vi "Get Hardware Channel Data (Rx or Tx).vi"(7 "direction":T11, 8 "error in":errorcluster, 11 "custom device ref in":T9 format="%.0x") -> (0 "error out":errorcluster, 2 "hardware channel data":T1[](array[typedef]) {"labels settings for RT"."Label Timestamp Channel Data Reference" format="%.0x"; "labels settings for RT"."Word Initial Raw Value" format="%032.0f"; "labels settings for RT"."Label Disable/Trigger Channel Reference" format="%.0x"; "labels settings for RT"."parameter driver data"."Tx parameter refs" format="%.0x"; "labels settings for RT"."parameter driver data"."Rx block data refs"."Data Reference" format="%.0x"; "labels settings for RT"."SDI" format="%02b"; "labels settings for RT"."label" format="%.0o"}, 3 "custom device ref out":T9 format="%.0x")   [LabVIEW 2020, in "Ballard ARINC 429 Shared.lvlib"]
uses:
  Ballard ARINC 429 Shared.lvlib
  <vilib>/NI VeriStand/Custom Device API/Custom Device API.lvlib
  Custom Device Support/Scripting/Communication Bus Template Scripting.lvlib
  <vilib>/NI VeriStand/Custom Device Tools/Custom Device Utility Library/Custom Device Utility Library.lvlib
  Custom Device Support/Scripting/Constants.vi
  <vilib>/NI VeriStand/Custom Device Tools/Custom Device Utility Library/NI VeriStand - Search for Item by GUID.vi
  <vilib>/NI VeriStand/Custom Device API/Data Access Type.ctl
  <vilib>/NI VeriStand/Custom Device API/Custom Device Item Ref.ctl
  <vilib>/NI VeriStand/Custom Device Tools/Custom Device Utility Library/NI VeriStand - Search for All Items by GUID.vi
  Label.ctl
  Encoding and Decoding/Encoding.ctl
  Encoding and Decoding/Encoding and Decoding.lvlib
  Protocol/Implementations/ARINC429/Parameter Definition.ctl
  Protocol/Implementations/ARINC429/ARINC 429.lvclass
  <vilib>/NI VeriStand/Custom Device API/Data Reference.ctl
  <vilib>/NI VeriStand/Custom Device API/Block Data Reference.ctl
  RT Parameters.ctl
  Transfer Type.ctl
  RT Label Settings.ctl
  RT Hardware Channel Settings.ctl
  <vilib>/NI VeriStand/Custom Device API/Get Item Property (U16).vi
  Direction.ctl
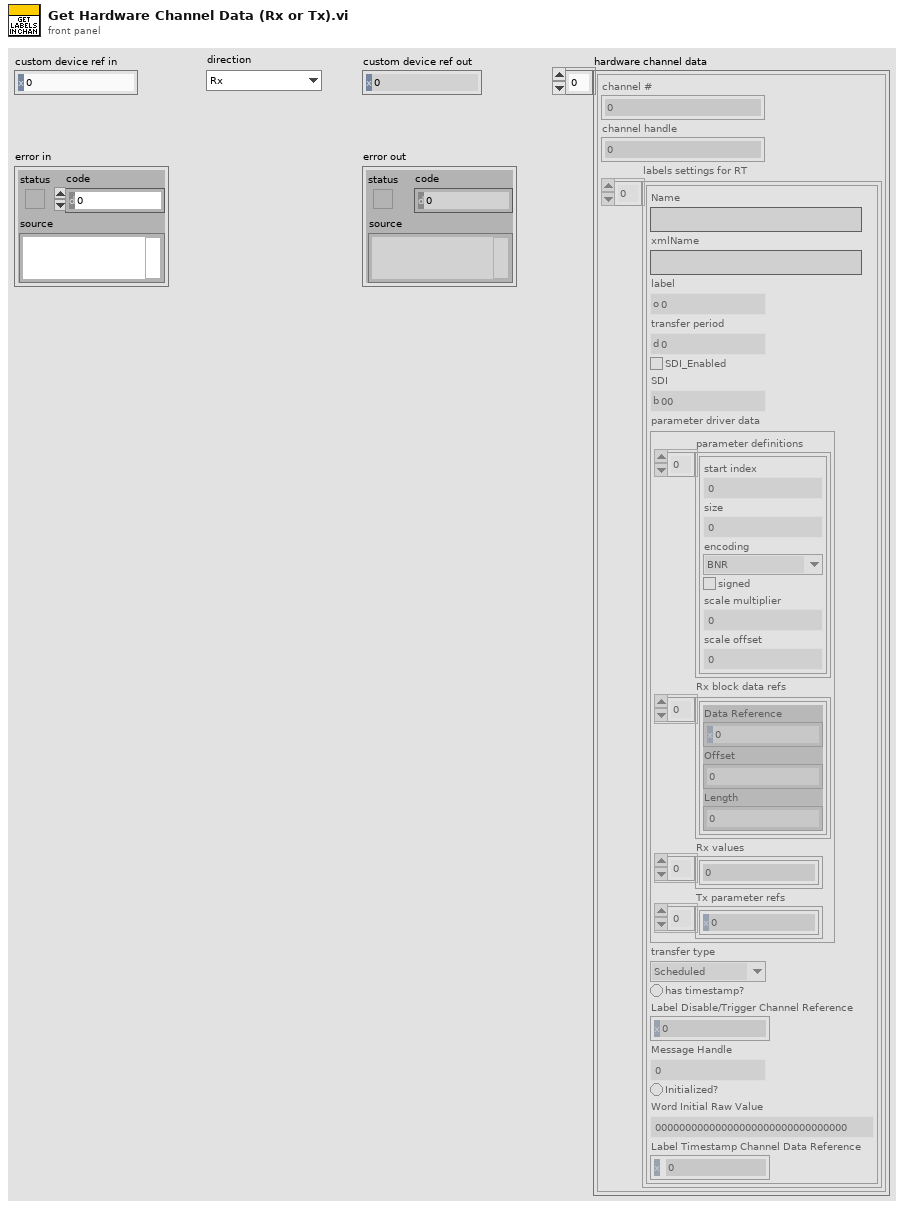
[diagram p1: front panel]
types:
  T1 = typedef "Ballard ARINC 429 Shared.lvlib/RT Hardware Channel Settings.ctl" = cluster{"channel #":u16, "channel handle":u64, "labels settings for RT":T2[]}
  T2 = typedef "Ballard ARINC 429 Shared.lvlib/RT Label Settings.ctl" = cluster{"Name":string, "xmlName":string, "label":T3, "transfer period":u32, "SDI_Enabled":bool, "SDI":u8, "parameter driver data":T4, "transfer type":T10, "has timestamp?":bool, "Label Disable/Trigger Channel Reference":T9, "Message Handle":u64, "Initialized?":bool, "Word Initial Raw Value":u32, "Label Timestamp Channel Data Reference":T8}
  T3 = typedef "Ballard ARINC 429 Shared.lvlib/Label.ctl" = u8
  T4 = typedef "Ballard ARINC 429 Shared.lvlib/RT Parameters.ctl" = cluster{"parameter definitions":T5[], "Rx block data refs":T7[], "Rx values":dbl[], "Tx parameter refs":T9[]}
  T5 = typedef "ARINC 429.lvclass/Parameter Definition.ctl" = cluster{"start index":i32, "size":i32, "encoding":T6, "signed":bool, "scale multiplier":dbl, "scale offset":dbl}
  T6 = typedef "Encoding and Decoding.lvlib/Encoding.ctl" = enum16{"BNR", "BCD", "Discrete"}
  T7 = typedef "Custom Device API.lvlib/Block Data Reference.ctl" = cluster{"Data Reference":T8, "Offset":u64, "Length":u64}
  T8 = typedef "Custom Device API.lvlib/Data Reference.ctl" = i32
  T9 = typedef "Custom Device API.lvlib/Custom Device Item Ref.ctl" = u64
  T10 = typedef "Ballard ARINC 429 Shared.lvlib/Transfer Type.ctl" = enum16{"Scheduled", "Acyclic", "Block", "Strobe"}
  T11 = typedef "Ballard ARINC 429 Shared.lvlib/Direction.ctl" = enum16{"Rx", "Tx"}
  T12 = typedef "Custom Device API.lvlib/Data Access Type.ctl" = enum16{"Read", "Write"}
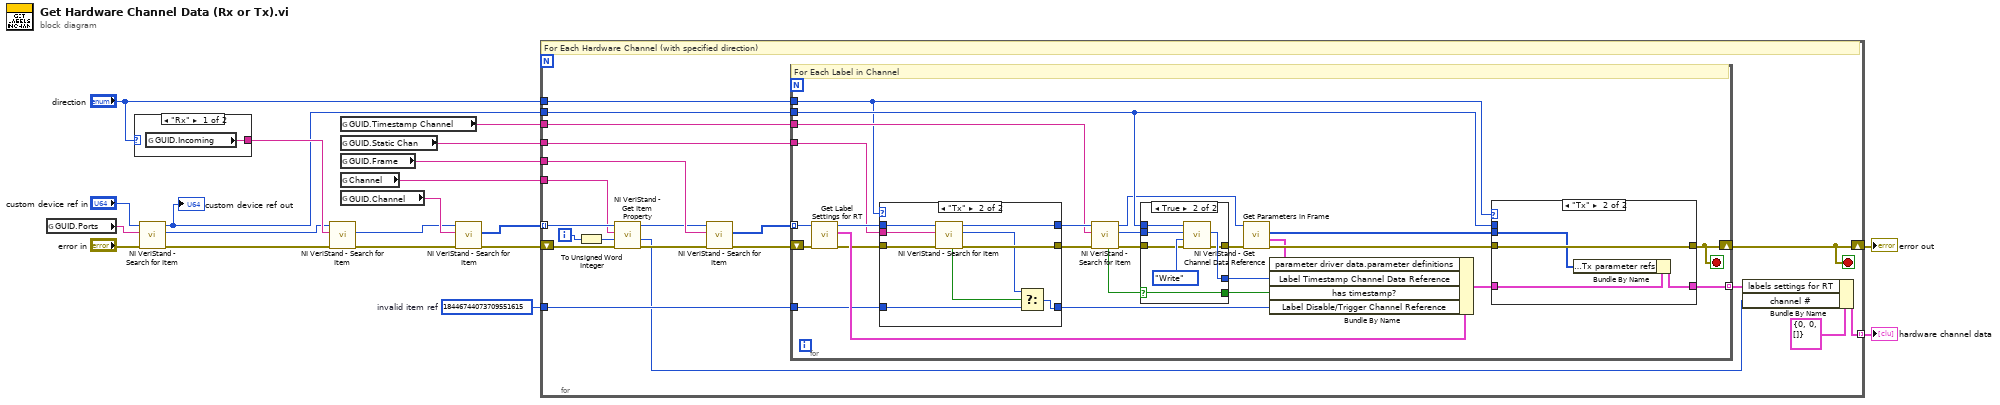
[diagram p0: block diagram]
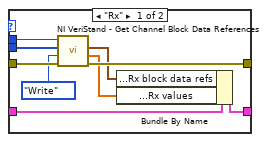
[diagram p4: hidden frame]
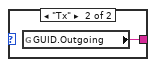
[diagram p5: hidden frame]
diagram:
  w10 = T9 18446744073709551615  # invalid item ref
  n1 = global read "Constants.vi" "GUID.Ports"() -> (w19:string)
  n2 = case shown="\"Rx\"" "direction" {
    tunnel: [w21 w22] -> w16
    frame "Rx" {
      n3 = global read "Constants.vi" "GUID.Incoming"() -> (w21:string)
    }
    frame "Tx" {
      n4 = global read "Constants.vi" "GUID.Outgoing"() -> (w22:string)
    }
  }
  n5 = call-poly <vilib>:"NI VeriStand - Search for Item.vi"("error in"="error in", "Item GUID"=w19, "Section Ref in"="custom device ref in") -> ("error out"=w14:errorcluster, "Item Ref"=w15:T9, "Section Ref out"=w3:T9)  [unwired: 5 in, 1 out]
  "custom device ref out" <- w3
  n6 = call-poly <vilib>:"NI VeriStand - Search for Item.vi"("error in"=w14, "Item GUID"=w16, "Section Ref in"=w15) -> ("error out"=w6:errorcluster, "Item Ref"=w7:T9)  [unwired: 5 in, 2 out]
  n7 = global read "Constants.vi" "GUID.Timestamp Channel"() -> (w11:string)
  n8 = global read "Constants.vi" "GUID.Static Chan"() -> (w12:string)
  n9 = global read "Constants.vi" "GUID.Frame"() -> (w20:string)
  n10 = global read "Constants.vi" "Channel"() -> (w2:string)
  n11 = global read "Constants.vi" "GUID.Channel"() -> (w8:string)
  n12 = call-poly <vilib>:"NI VeriStand - Search for Item.vi"("error in"=w6, "Item GUID"=w8, "Section Ref in"=w7) -> ("error out"=w5:errorcluster, "Item Refs"=w4:T9[])  [unwired: 5 in, 2 out]
  n13 = for {
    tunnel: w20 -> [w42]
    tunnel: w3 -> [w39]
    tunnel: "direction" -> [w38]
    tunnel: w12 -> [w37]
    tunnel: w11 -> [w36]
    tunnel: w10 -> [w35]
    shift-right: [w29] -> w9
    shift-left: w5 -> [w33]
    tunnel: w4 -> [w34] mode=indexing
    tunnel: w2 -> [w30]
    tunnel: [w26] -> w1 mode=indexing
    i -> [w28]
    stop <- w29 stop-if-true
    # "For Each Hardware Channel (with specified direction)"
    n14 = To Unsigned Word Integer(number=w28) -> (unsigned 16bit integer=w27:u16)
    n15 = call-poly <vilib>:"NI VeriStand - Get Item Property.vi"("error in (no error)"=w33, "Default Value"=w27, "Property Name"=w30, "Item Ref in"=w34) -> ("error out"=w31:errorcluster, "Value"=w24:u16, "Item Ref out"=w32:T9)  [unwired: 4 in, 1 out]
    n16 = call-poly <vilib>:"NI VeriStand - Search for Item.vi"("error in"=w31, "Item GUID"=w42, "Section Ref in"=w32) -> ("error out"=w40:errorcluster, "Item Refs"=w41:T9[])  [unwired: 5 in, 2 out]
    n17 = for {
      tunnel: w41 -> [w67] mode=indexing
      tunnel: w39 -> [w55]
      tunnel: w38 -> [w46]
      tunnel: w37 -> [w57]
      tunnel: w36 -> [w56]
      tunnel: w35 -> [w45]
      shift-right: [w43] -> w29
      shift-left: w40 -> [w66]
      tunnel: [w44] -> w25 mode=indexing
      stop <- w43 stop-if-true
      # "For Each Label in Channel"
      n18 = call "Get Label Settings for RT.vi"("error in"=w66, "label ref in"=w67) -> ("error out"=w61:errorcluster, "label settings for RT"=w64:T2, "Item Ref out"=w60:T9)  [unwired: 7 in]
      n19 = case shown="\"Tx\"" w46 {
        tunnel: w61 -> [w69 w80]
        tunnel: w60 -> [w70 w79]
        tunnel: [w70 w78] -> w59
        tunnel: [w69 w77] -> w58
        tunnel: w57 -> [_ w76]
        tunnel: [w71 w72] -> w47
        tunnel: w45 -> [w71 w74]
        frame "Rx", Default {
        }
        frame "Tx" {
          n20 = call-poly <vilib>:"NI VeriStand - Search for Item.vi"("error in"=w80, "Item GUID"=w76, "Section Ref in"=w79) -> ("error out"=w77:errorcluster, "Item Ref"=w73:T9, "Section Ref out"=w78:T9, "Found"=w75:bool)  [unwired: 5 in]
          n21 = Select(t=w73, s=w75, f=w74) -> (s? t:f=w72:T9)
        }
      }
      n22 = call-poly <vilib>:"NI VeriStand - Search for Item.vi"("error in"=w58, "Item GUID"=w56, "Section Ref in"=w59) -> ("error out"=w52:errorcluster, "Item Ref"=w54:T9, "Section Ref out"=w50:T9, "Found"=w49:bool)  [unwired: 5 in]
      n23 = case shown="True" w49 {
        selector: w49 -> [w81 w83]
        tunnel: w55 -> [_ w88]
        tunnel: w54 -> [_ w87]
        tunnel: [_ w86] -> w53
        tunnel: w52 -> [w82 w85]
        tunnel: [w82 w84] -> w51
        tunnel: [w81 w83] -> w48
        frame False {
        }
        frame True {
          n24 = call <vilib>:"NI VeriStand - Get Channel Data Reference.vi"("error in (no error)"=w85, "Access"=Data_Access_Type."Write", "Channel Ref in"=w87, "Device Ref in"=w88) -> ("error out"=w84:errorcluster, "Channel Data Reference"=w86:T8)  [unwired: 5 in, 1 out]
        }
      }
      n25 = call "Get Parameters in Frame.vi"("error in"=w51, "frame ref in"=w50) -> ("error out"=w65:errorcluster, "parameter definitions"=w63:T5[], "parameter references"=w68:T9[])  [unwired: 6 in, 1 out]
      n26 = Bundle By Name(cluster=w64, "parameter driver data.parameter definitions"=w63, "Label Timestamp Channel Data Reference"=w53, "has timestamp?"=w48, "Label Disable/Trigger Channel Reference"=w47) -> (w62:T2)
      n27 = case shown="\"Tx\"" w46 {
        tunnel: w68 -> [w98 w101]
        tunnel: w55 -> [w97 _]
        tunnel: w65 -> [w96 w102]
        tunnel: [w95 w102] -> w43
        tunnel: w62 -> [w92 w100]
        tunnel: [w91 w99] -> w44
        frame "Rx" {
          n28 = call <vilib>:"NI VeriStand - Get Channel Block Data References.vi"("error in (no error)"=w96, "Access"=Data_Access_Type."Write", "Channel Refs"=w98, "Device Ref in"=w97) -> ("error out"=w95:errorcluster, "Values Array"=w93:dbl[], "Block Data Refs"=w94:T7[])  [unwired: 4 in, 1 out]
          n29 = Bundle By Name(cluster=w92, "parameter driver data.Rx block data refs"=w94, "parameter driver data.Rx values"=w93) -> (w91:T2)
        }
        frame "Tx" {
          n30 = Bundle By Name(cluster=w100, "parameter driver data.Tx parameter refs"=w101) -> (w99:T2)
        }
      }
    }
    n31 = Bundle By Name(cluster=T1 {"channel #"=0, "channel handle"=0, "labels settings for RT"=[]} ("RT hardware channel"), "labels settings for RT"=w25, "channel #"=w24) -> (w26:T1)
  }
  "error out" <- w9
  "hardware channel data" <- w1
